vi "RectRegionConstraint_getMinMaxAccel.vi"(8 "Velocity_M/S":dbl, 9 "Curvature":dbl, 10 "statePose":T5={"TRANSLATION"={"X"=0.0, "Y"=0.0}, "ROTATION"={"VALUE"=0.0, "COS"=1.0, "SIN"=0.0}} {"ROTATION"."SIN" format="%13.4f"; "ROTATION"."COS" format="%13.4f"; "ROTATION"."VALUE" format="%13.4f"; "TRANSLATION"."Y" format="%14.3f"; "TRANSLATION"."X" format="%14.3f"}, 11 "RECT REGION CONSTRAINT":T1={"BottomLeftPoint"={"X"=0.0, "Y"=0.0}, "TopRightPoint"={"X"=0.0, "Y"=0.0}, "Constraint"=variant, "Constraint Type"=enum."DIFF DRIVE KINEMATICS"} {"TopRightPoint"."Y" format="%14.3f"; "TopRightPoint"."X" format="%14.3f"; "BottomLeftPoint"."Y" format="%14.3f"; "BottomLeftPoint"."X" format="%14.3f"}) -> (3 "TRAJ_CONSTAINT_MIN_MAX":T4)   [LabVIEW 2019, in "Trajectory_Library.lvlib"]
doc: "Return the minimum and maximum allowed acceleration given the provided conditions.\n\nIt appears that this routine doesn't do anything. It returns default values.\n\nParameters:\n - RectRegionConstraint - Constraint data structure\n - statePose - current traj state Pose\n - curvature - current traj curvature\n - maxVelocity - current traj max velocity\n\nReturns\n - TrajConstraint_Min_Max - Data structure with Min / Max acceleration."
uses:
  Trajectory_Library.lvlib
  TypeDef/POSE2D.ctl
  TypeDef/TRANSLATION2D.ctl
  TypeDef/ROTATION2D.ctl
  TypeDef/TRAJ_CONSTRAINT_MINMAX.ctl
  TypeDef/TRAJ_CONSTRAINT_RECT_REGION.ctl
  Enum/TRAJ_CONSTRAINT_TYPES_ENUM.ctl
  Pose2d_getXY.vi
  Translation2d_GetXY.vi
  MaxVelocityConstraint_getMinMaxAccel.vi
  DiffDriveKinematicsConstraint_getMinMaxAccel.vi
  DiffDriveVoltageConstraint_getMinMaxAccel.vi
  CentripetalAccelConstraint_getMinMaxAccel.vi
  MecaDriveKinematicsConstraint_getMinMaxAccel.vi
  SwerveDriveKinematicsConstraint_getMinMaxAccel.vi
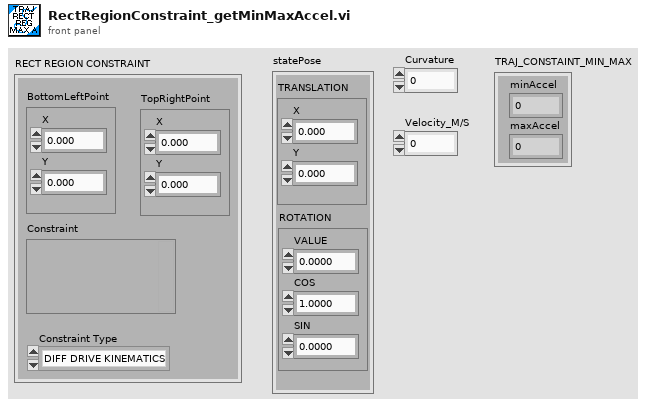
[diagram p1: front panel]
types:
  T1 = typedef "Trajectory_Library.lvlib/TRAJ_CONSTRAINT_RECT_REGION.ctl" = cluster{"BottomLeftPoint":T2, "TopRightPoint":T2, "Constraint":variant, "Constraint Type":T3}
  T2 = typedef "Trajectory_Library.lvlib/TRANSLATION2D.ctl" = cluster{"X":dbl, "Y":dbl}
  T3 = typedef "Trajectory_Library.lvlib/TRAJ_CONSTRAINT_TYPES_ENUM.ctl" = enum16{"UNDEFINED", "DIFF DRIVE KINEMATICS", "DIFF DRIVE VOLTAGE", "CENTRIPITAL ACCEL", "MECA DRIVE KINEMATICS", "SWERVE DRIVE KINEMATICS", "MAXIMUM VELOCITY", "ELLIPTICAL REGION", "RECTANGULAR REGION"}
  T4 = typedef "Trajectory_Library.lvlib/TRAJ_CONSTRAINT_MINMAX.ctl" = cluster{"minAccel":dbl, "maxAccel":dbl}
  T5 = typedef "Trajectory_Library.lvlib/POSE2D.ctl" = cluster{"TRANSLATION":T2, "ROTATION":T6}
  T6 = typedef "Trajectory_Library.lvlib/ROTATION2D.ctl" = cluster{"VALUE":dbl, "COS":dbl, "SIN":dbl}
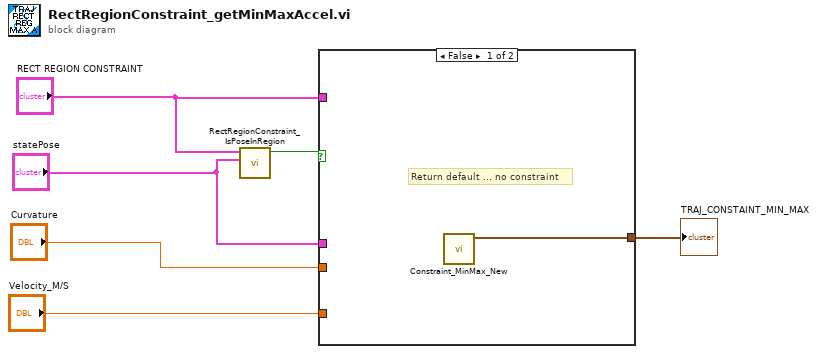
[diagram p0: block diagram]
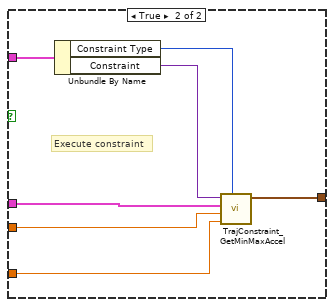
[diagram p2: hidden frame]
diagram:
  n1 = call "RectRegionConstraint_IsPoseInRegion.vi"("statePose"="statePose", "RECT_REGION_CONSTRAINT"="RECT REGION CONSTRAINT") -> ("PoseInRegion"=w6:bool)  [unwired: 9 in]
  n2 = case shown="False" w6 {
    tunnel: "RECT REGION CONSTRAINT" -> [_ w14]
    tunnel: "statePose" -> [_ w11]
    tunnel: "Curvature" -> [_ w10]
    tunnel: "Velocity_M/S" -> [_ w9]
    tunnel: [w7 w8] -> w1
    frame False {
      # "Return default ... no constraint"
      n3 = call "Constraint_MinMax_New.vi"() -> ("TRAJ_CONSTAINT_MIN_MAX"=w7:T4)  [unwired: 11 in]
    }
    frame True {
      # "Execute constraint"
      n4 = Unbundle By Name(w14) -> ("Constraint Type"=w13:T3, "Constraint"=w12:variant)
      n5 = call "TrajConstraint_GetMinMaxAccel.vi"("TrajjectoryConstraintType"=w13, "Velocity"=w9, "Curvature"=w10, "Pose"=w11, "Trajectory Constraint"=w12) -> ("Min Max Accel"=w8:T4)  [unwired: 6 in]
    }
  }
  "TRAJ_CONSTAINT_MIN_MAX" <- w1
